vi "Open Packets TDMS File.vi"(0 "serial input channel":string, 5 "base tdms file path":path, 7 "file operation type":T1(ring)=enum."open (read-only)", 11 "error in":errorcluster) -> (4 "packets file ref":refnum<k34>, 15 "error out":errorcluster)   [LabVIEW 2023, in "GettingStarted_Common_148X_Host.lvlib"]
uses:
  GettingStarted_Common_148X_Host.lvlib
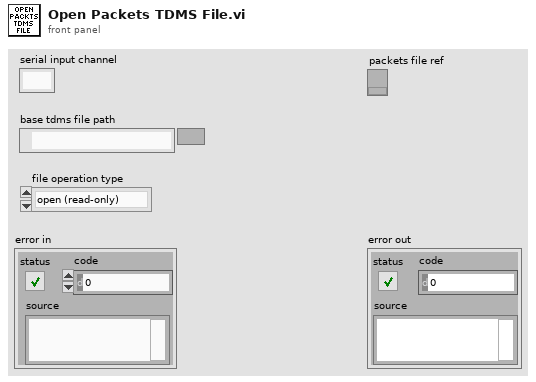
[diagram p1: front panel]
types:
  T1 = enum16{"open", "open or create", "create or replace", "create", "open (read-only)"}
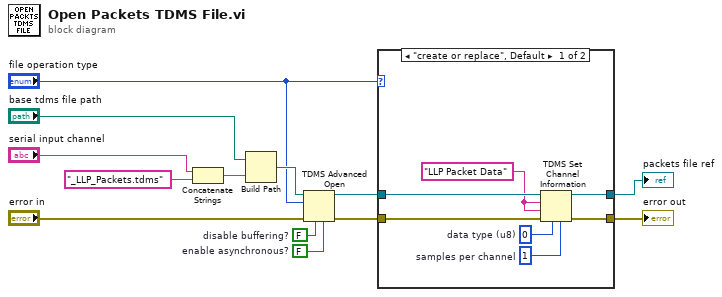
[diagram p0: block diagram]
diagram:
  w9 = FALSE  # enable asynchronous?
  w10 = FALSE  # disable buffering?
  n1 = Concatenate Strings("serial input channel", "_LLP_Packets.tdms") -> (w13:string)
  n2 = Build Path(base path="base tdms file path", name or relative path=w13) -> (appended path=w12:path)
  n3 = TDMS Advanced Open(4:w9, 6:w10, 8:"error in", 10:"file operation type", 11:w12) -> (0:w4:errorcluster, 3:w5:refnum<k34>)  [unwired: 1 out]
  n4 = case shown="\"create or replace\", Default" "file operation type" {
    tunnel: w5 -> [w18 w22]
    tunnel: [w15 w22] -> w2
    tunnel: w4 -> [w17 w21]
    tunnel: [w16 w21] -> w1
    frame "create or replace", Default {
      w14 = "LLP Packet Data" ("channel and group name")
      w20 = u32 1  # samples per channel
      w19 = u8 0  # data type (u8)
      n5 = TDMS Set Channel Information(4:w20, 6:w19, 8:w17, 9:w14, 10:w14, 11:w18) -> (0:w16:errorcluster, 3:w15:refnum<k34>)  [unwired: 1 in]
    }
    frame "open (read-only)" {
    }
  }
  "packets file ref" <- w2
  "error out" <- w1
